vi "HW_GEN - Parse VCH Physical Channel Info.vi"(8 "error in":errorcluster) -> (0 "error out":errorcluster)   [LabVIEW 2016]
uses:
  Ctrls/HardWare _ Module Configuration.ctl
panel:
  in  "Cfg in":T1[](array[typedef])
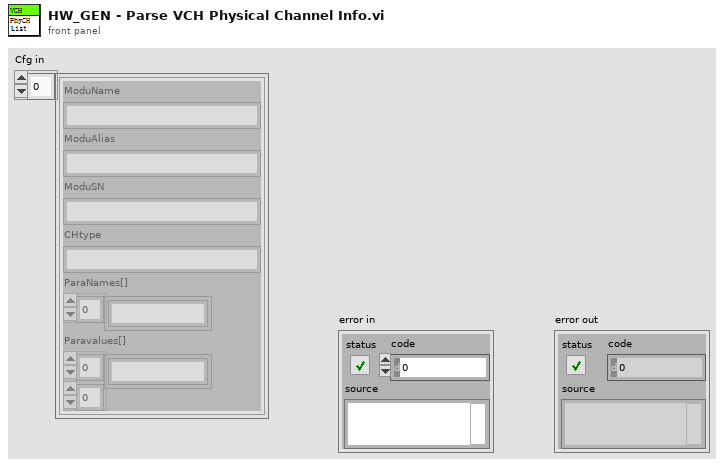
[diagram p1: front panel]
types:
  T1 = typedef "HardWare _ Module Configuration.ctl" = cluster{"ModuName":string, "ModuAlias":string, "ModuSN":string, "CHtype":string, "ParaNames[]":string[], "Paravalues[]":string[][]}
  T2 = cluster{"Left Cell String":string, "Child Text":string[], "Child Tag":string, "Item Indent":i32, "Child Only?":bool, "Glyph Index":i32}
  T3 = cluster{"Left Cell String":string, "Child Text":string[], "Child Tag":string, "Item Indent":i32, "Child Only?":bool, "Glyph Index":i32}[]
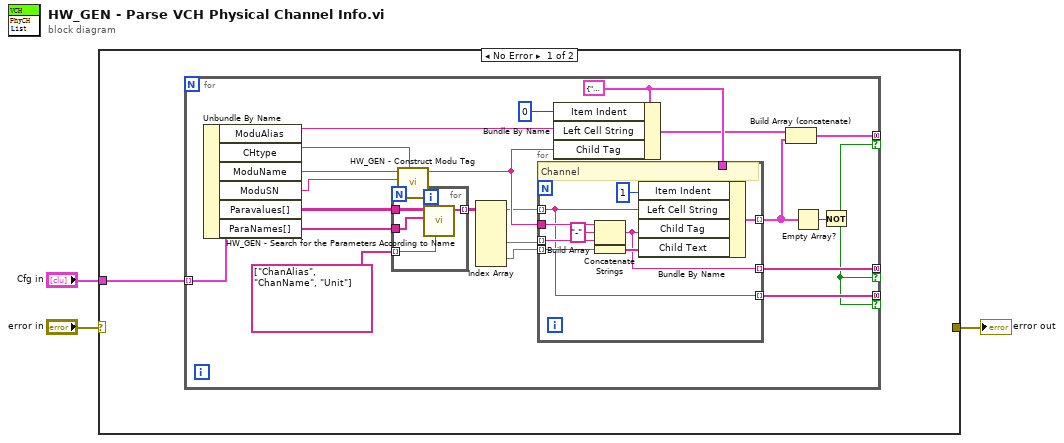
[diagram p0: block diagram]
diagram:
  n1 = case shown="No Error" "error in" {
    selector: "error in" -> [_ w41]
    tunnel: [_ w41] -> w2
    tunnel: "Cfg in" -> [w4 _]
    frame No Error {
      n2 = for {
        tunnel: w4 -> [w26] mode=indexing
        tunnel: [w8] -> _ mode=concatenating if=w5
        tunnel: [w7] -> _ mode=concatenating if=w5
        tunnel: [w6] -> _ mode=concatenating if=w5
        w20 = T2 {"Left Cell String"="", "Child Text"=[], "Child Tag"="", "Item Indent"=0, "Child Only?"=FALSE, "Glyph Index"=0} ("Item")
        n3 = Unbundle By Name(w26) -> ("ModuAlias"=w25:string, "CHtype"=w24:string, "ModuName"=w23:string, "ModuSN"=w22:string, "Paravalues[]"=w17:string[][], "ParaNames[]"=w16:string[])
        n4 = for {
          tunnel: w17 -> [w29]
          tunnel: w16 -> [w28]
          tunnel: [w30] -> w19 mode=indexing
          tunnel: string[] ["ChanAlias", "ChanName", "Unit"] ("ParaNames[]") -> [w27] mode=indexing
          n5 = call "HW_GEN - Search for the Parameters According to Name.vi"("ParaName"=w27, "ParaNames[]"=w28, "Paravalues[] in"=w29) -> ("Paravalues[] out"=w30:string[])  [unwired: 8 in]
        }
        n6 = call "HW_GEN - Construct Modu Tag.vi"("ChanType"=w24, "ModSN"=w22, "ModName"=w23) -> ("String"=w18:string)  [unwired: 8 in]
        n7 = Index Array(array=w19) -> (element #1=w14:string[], element #2=w13:string[], element #3=w12:string[])  [unwired: 6 in]
        n8 = for {
          tunnel: w14 -> [w31] mode=indexing
          tunnel: w20 -> [w40]
          tunnel: [w39] -> w9 mode=indexing
          tunnel: w13 -> [w35] mode=indexing
          tunnel: w12 -> [w37] mode=indexing
          tunnel: w18 -> [w36]
          tunnel: [w32] -> w7 mode=indexing
          tunnel: [w31] -> w6 mode=indexing
          # "Channel"
          n9 = Concatenate Strings(w36, "-" ("string"), w35) -> (w32:string)
          n10 = Build Array(w37) -> (w38:string[])
          n11 = Bundle By Name(cluster=w40, "Item Indent"=1, "Left Cell String"=w31, "Child Tag"=w32, "Child Text"=w38) -> (w39:T2)
        }
        n12 = Bundle By Name(cluster=w20, "Item Indent"=0, "Left Cell String"=w25, "Child Tag"=w18) -> (w10:T2)
        n13 = Build Array (concatenate)(w10, w9) -> (w8:T3)
        n14 = Empty Array?(array=w9) -> (empty?=w11:bool)
        n15 = Not(x=w11) -> (.not. x?=w5:bool)
      }
    }
    frame Error {
    }
  }
  "error out" <- w2
